vi "AH_READ2.VI"() -> ()   [LabVIEW 2021]
panel:
  in  "V excitation":T1(ring)
  in  "BIas":enum16{"Disabled", "100 MOhm", "1 MOhm"}(ring)
  in  "ALternate":enum16{"0", "1", "2", "3", "4", "5", "6", "7"}(ring)=enum."1"
  in  "AVerage":T2(ring)=enum."5"
  out "?":cluster{"capacitance":dbl, "loss":dbl}(graph)
  out "loss (nSiemens)":dbl format="%.8f"
  out "capacitance (pF)":dbl format="%.8f"
  in  "Read delay (ms)":u32=3000
  in  "AH2500A address":string="20"
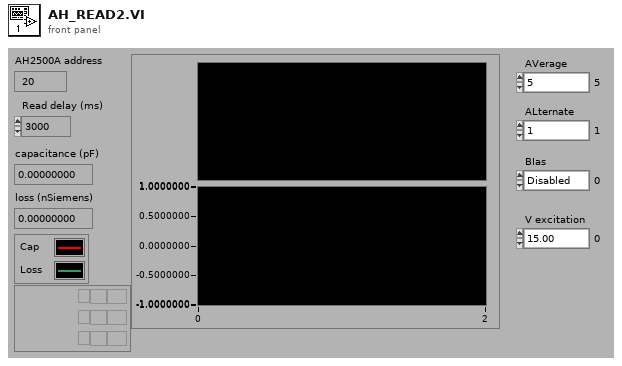
[diagram p1: front panel]
types:
  T1 = enum16{"15.00", "7.50", "3.75", "3.00", "1.50", "0.750", "0.375", "0.250", "0.125", "0.100", "0.050", "0.030", "0.015", "0.010", "0.0050", "0.0030", "0.0015", "0.0010", "0.0005"}
  T2 = enum16{"0", "1", "2", "3", "4", "5", "6", "7", "8", "9", "10", "11", "12", "13", "14", "15"}
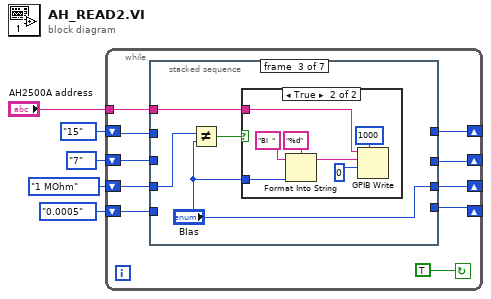
[diagram p0: block diagram]
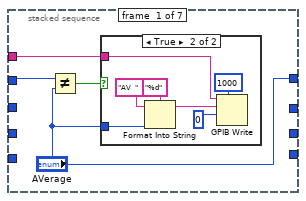
[diagram p2: hidden frame]
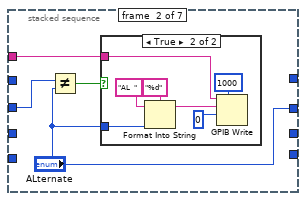
[diagram p4: hidden frame]
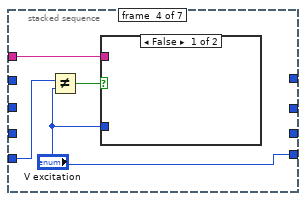
[diagram p7: hidden frame]
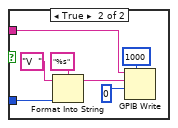
[diagram p8: hidden frame]
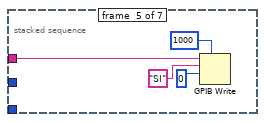
[diagram p9: hidden frame]
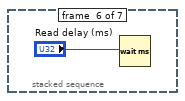
[diagram p10: hidden frame]
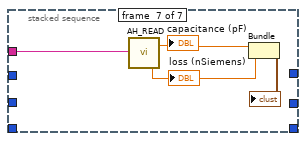
[diagram p11: hidden frame]
diagram:
  n1 = while {
    shift-left: T1."0.0005" ("V excitation") -> [w6]
    shift-right: [w7] -> _
    shift-left: enum16{"Disabled", "100 MOhm", "1 MOhm"}."1 MOhm" ("BIas") -> [w8]
    shift-right: [w9] -> _
    shift-left: enum16{"0", "1", "2", "3", "4", "5", "6", "7"}."7" ("ALternate") -> [w10]
    shift-right: [w11] -> _
    shift-left: T2."15" ("AVerage") -> [w13]
    shift-right: [w12] -> _
    tunnel: "AH2500A address" -> [w14]
    stop <- TRUE continue-if-true
    n2 = stacked-sequence {
      tunnel: w14 -> [w18 w30 w41 w52 w60 _ w68]
      tunnel: w13 -> [w19 _ _ _ _ _ _]
      tunnel: ["AVerage" _ _ _ _ _ _] -> w12
      tunnel: [_ "ALternate" _ _ _ _ _] -> w11
      tunnel: w10 -> [_ w27 _ _ _ _ _]
      tunnel: [_ _ "BIas" _ _ _ _] -> w9
      tunnel: w8 -> [_ _ w38 _ _ _ _]
      tunnel: [_ _ _ "V excitation" _ _ _] -> w7
      tunnel: w6 -> [_ _ _ w50 _ _ _]
      frame #0 {
        n3 = Not Equal?(x=w19, y="AVerage") -> (x != y?=w17:bool)
        n4 = case shown="True" w17 {
          tunnel: "AVerage" -> [_ w24]
          tunnel: w18 -> [_ w20]
          frame False {
          }
          frame True {
            n5 = Format Into String(format string="%d", initial string="AV  ", w24) -> (resulting string=w21:string)  [unwired: 1 in, 1 out]
            n6 = GPIB Write(0:w20, 1:w21, 2:i16 0, 4:1000 ("timeout ms (488.2 global)")) -> ()  [unwired: 1 in, 2 out]
          }
        }
      }
      frame #1 {
        n7 = Not Equal?(x=w27, y="ALternate") -> (x != y?=w29:bool)
        n8 = case shown="True" w29 {
          tunnel: "ALternate" -> [_ w35]
          tunnel: w30 -> [_ w31]
          frame False {
          }
          frame True {
            n9 = Format Into String(format string="%d", initial string="AL  ", w35) -> (resulting string=w32:string)  [unwired: 1 in, 1 out]
            n10 = GPIB Write(0:w31, 1:w32, 2:i16 0, 4:1000 ("timeout ms (488.2 global)")) -> ()  [unwired: 1 in, 2 out]
          }
        }
      }
      frame #2 {
        n11 = Not Equal?(x=w38, y="BIas") -> (x != y?=w40:bool)
        n12 = case shown="True" w40 {
          tunnel: "BIas" -> [_ w46]
          tunnel: w41 -> [_ w42]
          frame False {
          }
          frame True {
            n13 = Format Into String(format string="%d", initial string="BI  ", w46) -> (resulting string=w43:string)  [unwired: 1 in, 1 out]
            n14 = GPIB Write(0:w42, 1:w43, 2:i16 0, 4:1000 ("timeout ms (488.2 global)")) -> ()  [unwired: 1 in, 2 out]
          }
        }
      }
      frame #3 {
        n15 = Not Equal?(x=w50, y="V excitation") -> (x != y?=w51:bool)
        n16 = case shown="False" w51 {
          tunnel: "V excitation" -> [_ w57]
          tunnel: w52 -> [_ w53]
          frame False {
          }
          frame True {
            n17 = Format Into String(format string="%s", initial string="V  ", w57) -> (resulting string=w54:string)  [unwired: 1 in, 1 out]
            n18 = GPIB Write(0:w53, 1:w54, 2:i16 0, 4:1000 ("timeout ms (488.2 global)")) -> ()  [unwired: 1 in, 2 out]
          }
        }
      }
      frame #4 {
        n19 = GPIB Write(0:w60, 1:"SI", 2:i16 0, 4:1000 ("timeout ms (488.2 global)")) -> ()  [unwired: 1 in, 2 out]
      }
      frame #5 {
        n20 = Wait (ms)(milliseconds to wait="Read delay (ms)") -> ()  [unwired: 1 out]
      }
      frame #6 {
        n21 = call "AH_READ.VI"("AH2500A address"=w68) -> ("capacitance"=w65:dbl, "loss"=w67:dbl)
        "capacitance (pF)" <- w65
        "loss (nSiemens)" <- w67
        n22 = Bundle("capacitance"=w65, "loss"=w67) -> (→"?":cluster{"capacitance":dbl, "loss":dbl})  [unwired: 1 in]
      }
    }
  }
